vi "InitPluginPaths.vi"(8 "ErrorArray":errorcluster[](array[cluster]), 9 "PluginPathArray":string[](array[string]), 10 "RingRefArray":refnum<vi>[](array[refnum]), 11 "TestBase in":refnum<class "TestBase.lvclass">) -> (0 "ErrorArray":errorcluster[](array[cluster]), 3 "TestBase out":refnum<class "TestBase.lvclass">)   [LabVIEW 2014, in "TestBase.lvclass"]
uses:
  TestBase.lvclass
  TestBase.lvclass/TestBase.ctl
  Accessors/Write PluginPathArray.vi
  LV_Ini/Ini_lib.lvlib
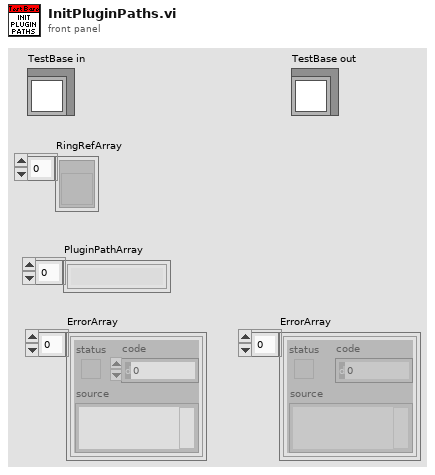
[diagram p1: front panel]
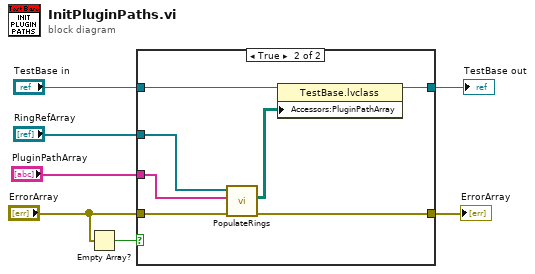
[diagram p0: block diagram]
diagram:
  n1 = Empty Array?(array="ErrorArray") -> (empty?=w4:bool)
  n2 = case shown="True" w4 {
    tunnel: [w9 w14] -> w3
    tunnel: [w8 w11] -> w6
    tunnel: "TestBase in" -> [w8 w16]
    tunnel: "ErrorArray" -> [w9 w15]
    tunnel: "PluginPathArray" -> [_ w13]
    tunnel: "RingRefArray" -> [_ w12]
    frame False {
    }
    frame True {
      n3 = call "PopulateRings.vi"("ErrorArray In"=w15, "RelativePathToIniArray"=w13, "RingRefArray"=w12) -> ("ErrorArray Out"=w14:errorcluster[], "INIFilePathsArray"=w10:path[][])  [unwired: 7 in]
      n4 = property class="TestBase.lvclass"(reference=w16, "Accessors:PluginPathArray"=w10) -> (reference out=w11:refnum<class "TestBase.lvclass">)  [unwired: 1 in, 1 out]
    }
  }
  "TestBase out" <- w6
  "ErrorArray" <- w3
